vi "Read AnchorID.vi"(0 "Anchor in":refnum<class "Anchor.lvclass">, 1 "error in (no error)":errorcluster) -> (2 "Anchor out":refnum<class "Anchor.lvclass">, 3 "AnchorID":dbl, 4 "error out":errorcluster)   [LabVIEW 2014, in "Anchor.lvclass"]
uses:
  Anchor.lvclass
  Anchor.lvclass/Anchor.ctl
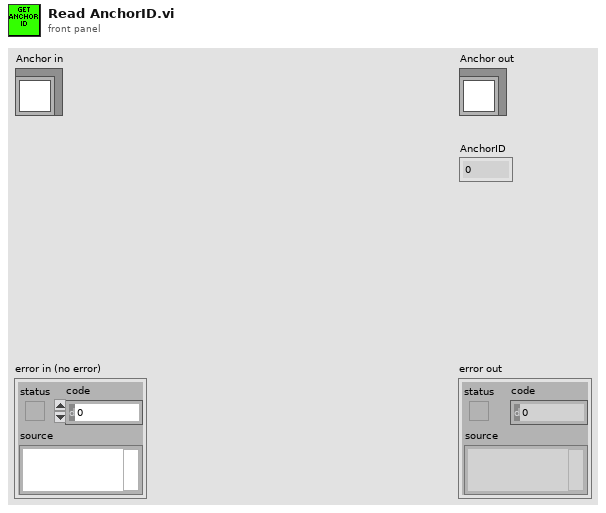
[diagram p1: front panel]
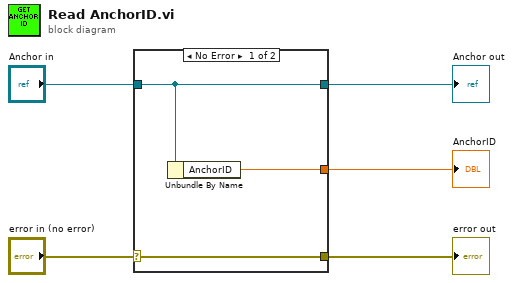
[diagram p0: block diagram]
diagram:
  n1 = case shown="No Error" "error in (no error)" {
    selector: "error in (no error)" -> [w8 w9]
    tunnel: [w8 w9] -> w4
    tunnel: [w7 w10] -> w2
    tunnel: "Anchor in" -> [w7 w10]
    tunnel: [w6 _] -> w1
    frame No Error {
      n2 = Unbundle By Name(w7) -> ("AnchorID"=w6:dbl)
    }
    frame Error {
    }
  }
  "error out" <- w4
  "Anchor out" <- w2
  "AnchorID" <- w1
